vi "Untitled 1.vi"() -> ()   [LabVIEW 2011]
panel:
  out "data string 2":string
  out "data string":string
  out "*(type *) &x":string
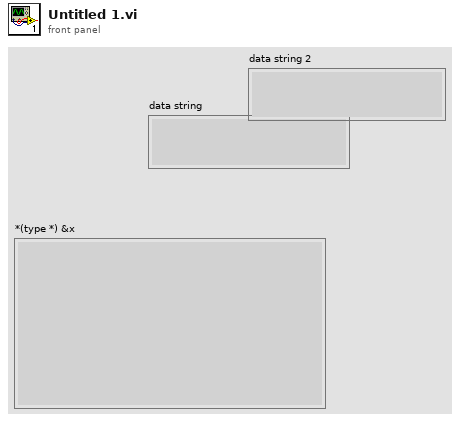
[diagram p1: front panel]
types:
  T1 = enum16{"big-endian, network order", "native, host order", "little-endian"}
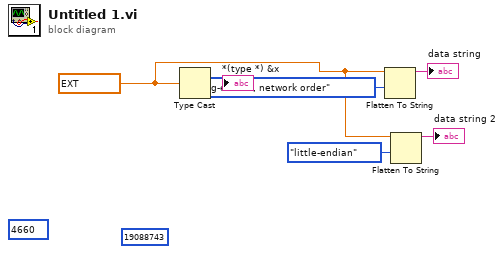
[diagram p0: block diagram]
diagram:
  (unwired) 4660
  (unwired) u32 19088743
  w4 = ext 12345678.0 ("x")
  n1 = Type Cast(x=w4) -> (*(type *) &x=→"*(type *) &x":string)  [unwired: 1 in]
  n2 = Flatten To String(anything=w4, byte order (0:big-endian, network order)=T1."big-endian, network order") -> (data string=→"data string":string)  [unwired: 2 in, 2 out]
  n3 = Flatten To String(anything=w4, byte order (0:big-endian, network order)=T1."little-endian") -> (data string=→"data string 2":string)  [unwired: 2 in, 2 out]
